vi "configureMode.vi"(8 "error in (no error)":errorcluster, 11 "ElectrometerController in":refnum<class "ElectrometerController.lvclass">) -> (0 "error out":errorcluster, 2 "Mode":T1, 3 "ElectrometerController out":refnum<class "ElectrometerController.lvclass">)   [LabVIEW 2016, in "ElectrometerController.lvclass"]
uses:
  ElectrometerController.lvclass
  Electrometer/Modes.ctl
  Electrometer/Electrometer.lvclass
  ElectrometerConfiguration/ElectrometerInternalConfiguration.lvclass
  Electrometer/State/ElectrometerState.lvclass
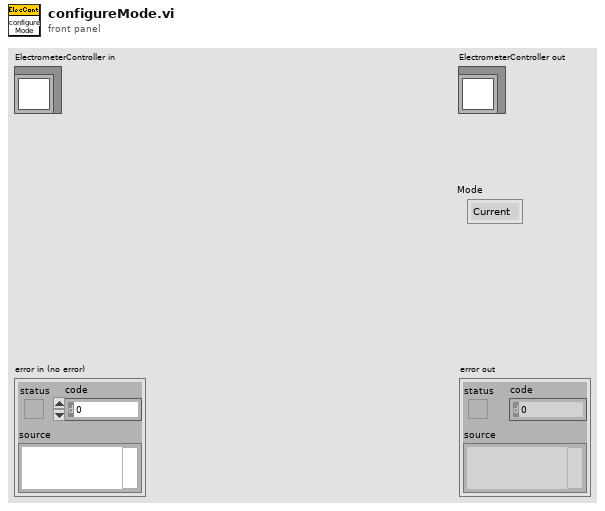
[diagram p1: front panel]
types:
  T1 = typedef "Electrometer.lvclass/Modes.ctl" = enum16{"Current", "Charge"}
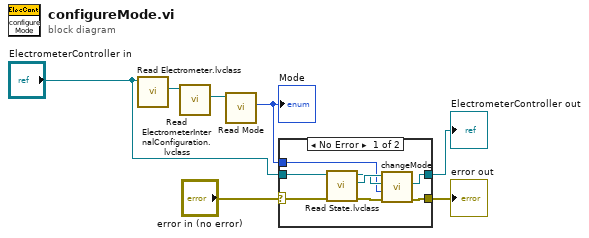
[diagram p0: block diagram]
diagram:
  n1 = call-dynamic "Read Electrometer.lvclass.vi"("ElectrometerController in"="ElectrometerController in") -> ("Electrometer.lvclass"=w4:refnum<class "Electrometer.lvclass">)  [unwired: 8 in, 2 out]
  n2 = call-dynamic "Read ElectrometerInternalConfiguration.lvclass.vi"("Electrometer in"=w4) -> ("ElectrometerInternalConfiguration.lvclass"=w5:refnum<class "ElectrometerInternalConfiguration.lvclass">)  [unwired: 8 in, 2 out]
  n3 = call-dynamic "Read Mode.vi"("ElectrometerInternalConfiguration in"=w5) -> ("Measurement Function (0: Current)"=w1:T1)  [unwired: 8 in, 2 out]
  "Mode" <- w1
  n4 = case shown="No Error" "error in (no error)" {
    selector: "error in (no error)" -> [w11 w17]
    tunnel: [w12 w17] -> w6
    tunnel: [w9 w16] -> w3
    tunnel: "ElectrometerController in" -> [w10 w16]
    tunnel: w1 -> [w8 _]
    frame No Error {
      n5 = call-dynamic "Read State.lvclass.vi"("error in (no error)"=w11, "ElectrometerController in"=w10) -> ("error out"=w15:errorcluster, "ElectrometerState"=w14:refnum<class "ElectrometerState.lvclass">, "ElectrometerController out"=w13:refnum<class "ElectrometerController.lvclass">)  [unwired: 7 in]
      n6 = call-dynamic "changeMode.vi"("error in (no error)"=w15, "Mode"=w8, "ElectrometerController in"=w13, "State in"=w14) -> ("error out"=w12:errorcluster, "ElectrometerController out"=w9:refnum<class "ElectrometerController.lvclass">)  [unwired: 5 in, 1 out]
    }
    frame Error {
    }
  }
  "error out" <- w6
  "ElectrometerController out" <- w3
